vi "createElement.vi"(6 "collectionInfo":T1, 8 "error in (no error)":errorcluster, 9 "elementBasicType":string, 10 "elementName":string, 11 "Topic in":refnum<class "Topic.lvclass">) -> (0 "error out":errorcluster, 3 "Topic out":refnum<class "Topic.lvclass">)   [LabVIEW 2018, in "Topic.lvclass"]
uses:
  Topic.lvclass
  Typedefs/CollectionInfo.ctl
  Topic.lvclass/Topic.ctl
  ElementFactory/IElementFactory/IElementFactory.lvclass
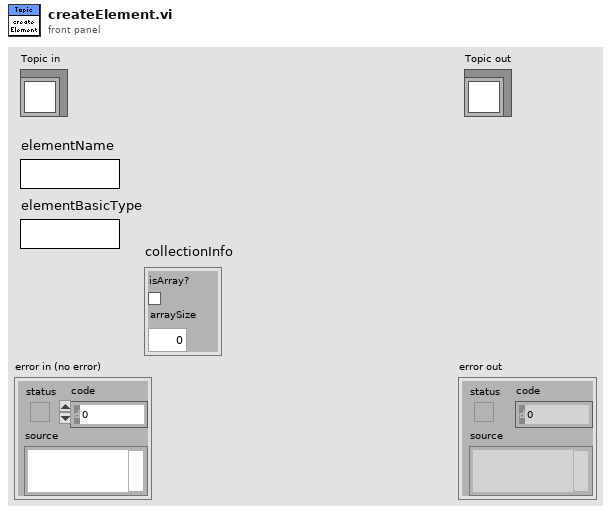
[diagram p1: front panel]
types:
  T1 = typedef "CollectionInfo.ctl" = cluster{"isArray?":bool, "arraySize":u16}
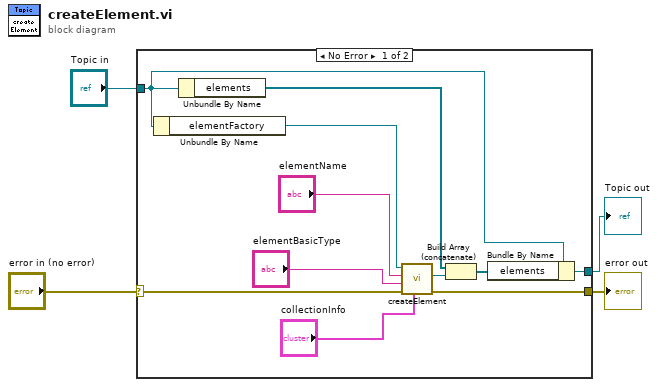
[diagram p0: block diagram]
diagram:
  n1 = case shown="No Error" "error in (no error)" {
    selector: "error in (no error)" -> [w11 w17]
    tunnel: [w10 w17] -> w3
    tunnel: [w8 w16] -> w1
    tunnel: "Topic in" -> [w9 w16]
    frame No Error {
      n2 = Unbundle By Name(w9) -> ("elementFactory"=w15:refnum<class "IElementFactory.lvclass">)
      n3 = Unbundle By Name(w9) -> ("elements"=w7:refnum<class "Element.lvclass">[])
      n4 = call-dynamic "createElement.vi"("collectionInfo"="collectionInfo", "error in (no error)"=w11, "elementBasicType"="elementBasicType", "elementName"="elementName", "IElementFactory in"=w15) -> ("error out"=w10:errorcluster, "element"=w6:refnum<class "Element.lvclass">)  [unwired: 4 in, 1 out]
      n5 = Build Array (concatenate)(w7, w6) -> (w5:refnum<class "Element.lvclass">[])
      n6 = Bundle By Name(cluster=w9, "elements"=w5) -> (w8:refnum<class "Topic.lvclass">)
    }
    frame Error {
    }
  }
  "error out" <- w3
  "Topic out" <- w1
